vi "Low_Power_CH1.vi"(8 "Modulation parameter":T1, 9 "output bits":i8[](array[numeric]), 10 "Boolean":bool, 11 "Record BER":bool) -> (3 "subarray":i8[](array[numeric]))   [LabVIEW 2022 SP3]
panel:
  out "No. Bits LP":dbl
  out "?":T1
  out "Low-Power Decoded Message":string
  in  "Expected message LP":string="Non Critical Data\nNon Critical Data\nNon Critical Data\nNon Critical Data\nNon Critical Data"
  out "Acum. Err LP":dbl
  out "Acc. BER LP":dbl format="%#_4g"
  out "Inst. BER LP":dbl format="%#_4g"
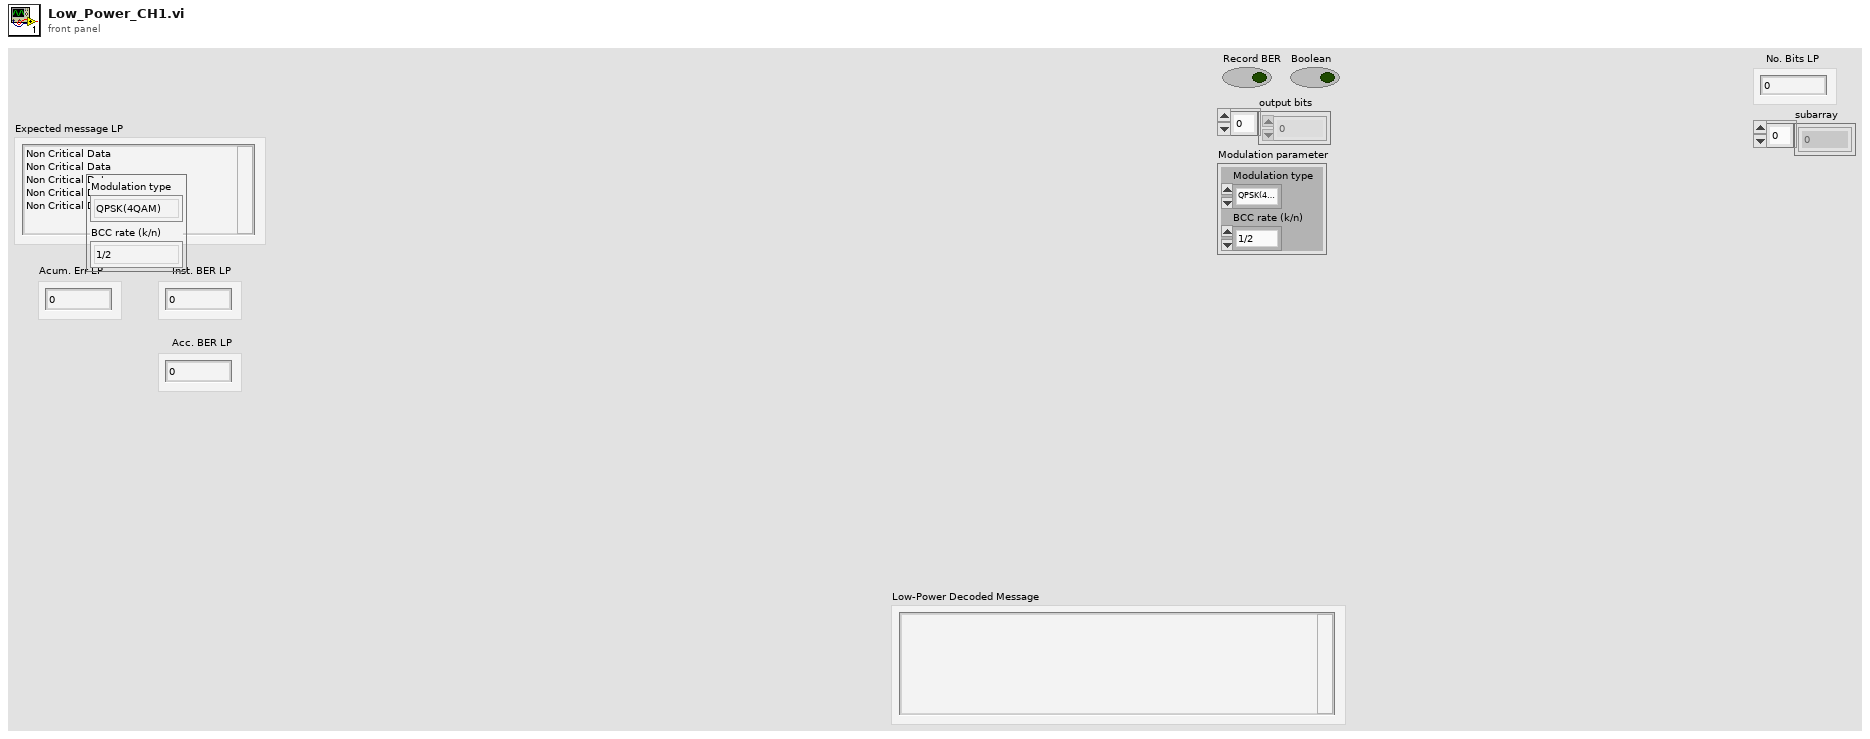
[diagram p1: front panel]
types:
  T1 = cluster{"Modulation type":enum16{"QPSK(4QAM)", "64QAM", "16QAM", "BPSK"}, "BCC rate (k/n)":enum16{"1/2", "2/3", "3/4"}}
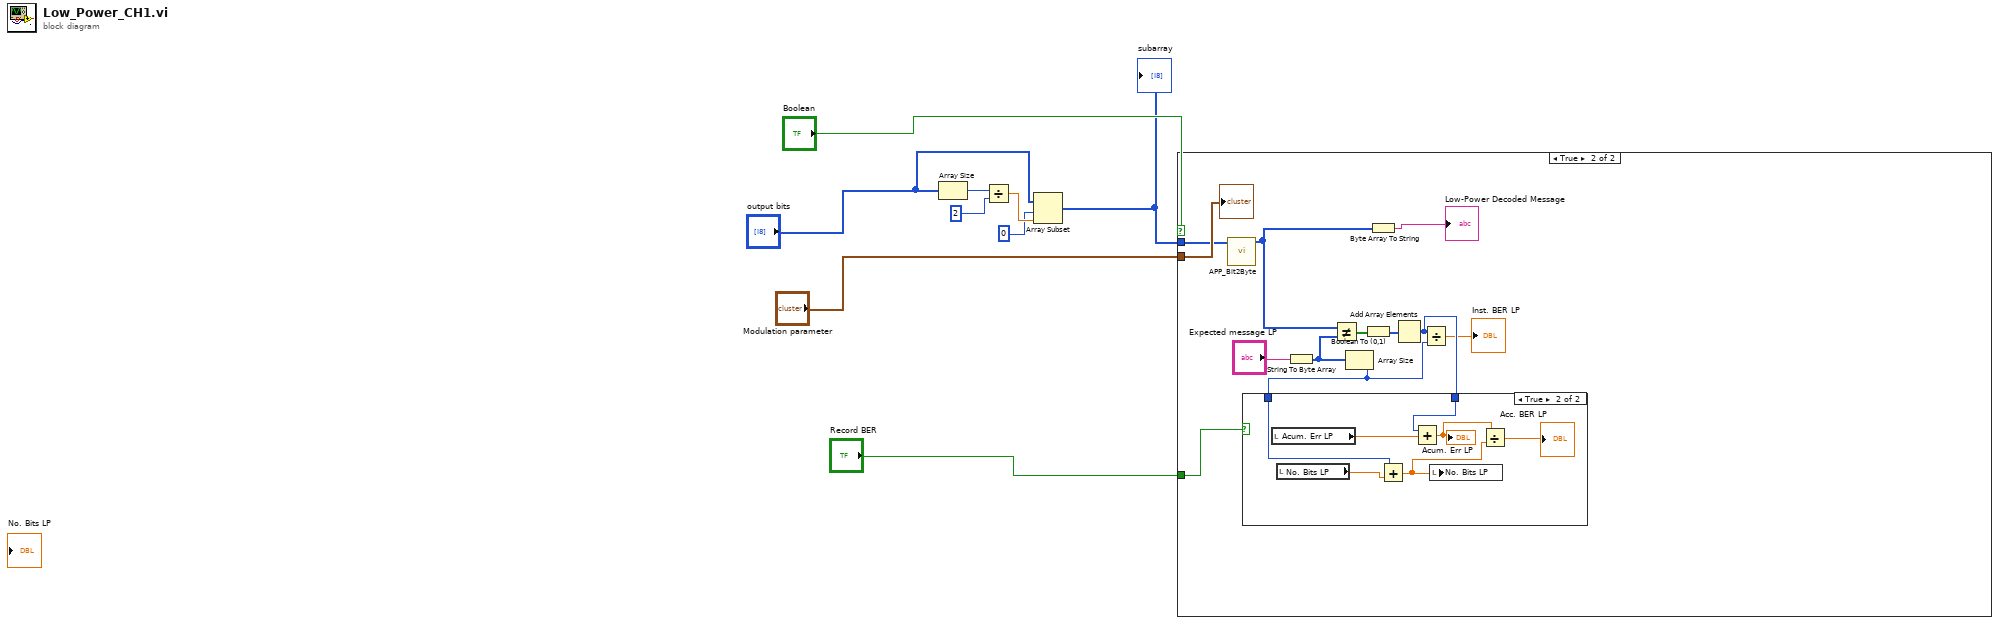
[diagram p0: block diagram]
diagram:
  n1 = Array Size(array="output bits") -> (size(s)=w6:i32)
  n2 = Divide(x=w6, y=2) -> (x/y=w4:dbl)
  n3 = Array Subset(array="output bits", index=0, length=w4) -> (w1:i8[])
  "subarray" <- w1
  n4 = case shown="True" "Boolean" {
    tunnel: "Modulation parameter" -> [_ w21]
    tunnel: "Record BER" -> [_ w12]
    tunnel: w1 -> [_ w10]
    frame False {
    }
    frame True {
      n5 = call "APP_Bit2Byte.vi"("input bit stream"=w10) -> ("output byte stream"=w14:u8[])  [unwired: 10 in]
      n6 = String To Byte Array(string="Expected message LP") -> (unsigned byte array=w18:u8[])
      n7 = Not Equal?(x=w14, y=w18) -> (x != y?=w16:bool[])
      n8 = Array Size(array=w18) -> (size(s)=w19:i32)
      n9 = Boolean To (0,1)(Boolean=w16) -> (0, 1=w15:i16[])
      n10 = Byte Array To String(unsigned byte array=w14) -> (string=→"Low-Power Decoded Message":string)
      n11 = Add Array Elements(numeric array=w15) -> (sum=w13:i16)
      n12 = case shown="True" w12 {
        tunnel: w19 -> [_ w27]
        tunnel: w13 -> [_ w25]
        frame False {
        }
        frame True {
          n13 = local read "Acum. Err LP"() -> (w26:dbl)
          n14 = local read "No. Bits LP"() -> (w28:dbl)
          n15 = Add(x=w27, y=w28) -> (x+y=w22:dbl)
          n16 = Add(x=w25, y=w26) -> (x+y=w24:dbl)
          "Acum. Err LP" <- w24
          n17 = local write "No. Bits LP"(w22) -> ()
          n18 = Divide(x=w24, y=w22) -> (x/y=→"Acc. BER LP":dbl)
        }
      }
      n19 = Divide(x=w13, y=w19) -> (x/y=→"Inst. BER LP":dbl)
      "?" <- w21
    }
  }
